vi "Инвертирование знака числа(5-разрядного)v2.vi"(1 "sign":bool, 2 "A":T2) -> (0 "R":T1)   [LabVIEW 2013]
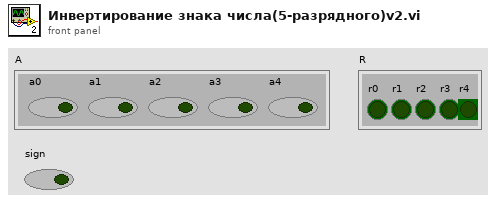
[diagram p1: front panel]
types:
  T1 = cluster{"r0":bool, "r1":bool, "r2":bool, "r3":bool, "r4":bool}
  T2 = cluster{"a0":bool, "a1":bool, "a2":bool, "a3":bool, "a4":bool}
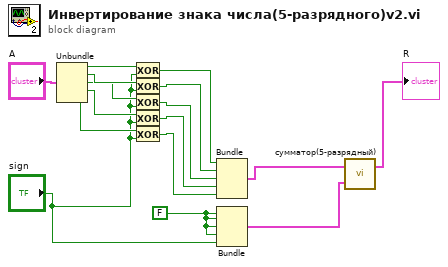
[diagram p0: block diagram]
diagram:
  w2 = FALSE
  n1 = Unbundle("A") -> ("a0"=w3:bool, "a1"=w15:bool, "a2"=w14:bool, "a3"=w13:bool, "a4"=w12:bool)
  n2 = Exclusive Or(1:"sign", 2:w3) -> (0:w8:bool)
  n3 = Exclusive Or(1:"sign", 2:w15) -> (0:w7:bool)
  n4 = Exclusive Or(1:"sign", 2:w14) -> (0:w6:bool)
  n5 = Exclusive Or(1:"sign", 2:w13) -> (0:w5:bool)
  n6 = Exclusive Or(1:"sign", 2:w12) -> (0:w4:bool)
  n7 = Bundle(w8, w7, w6, w5, w4) -> (w11:cluster{bool, bool, bool, bool, bool})  [unwired: 1 in]
  n8 = Bundle(w2, w2, w2, w2, "sign"="sign") -> (w10:cluster{bool, bool, bool, bool, "sign":bool})  [unwired: 1 in]
  n9 = call "сумматор(5-разрядный).vi"("B"=w10, "A"=w11) -> ("R"=→"R":T1)  [unwired: 1 out]
